vi "SUMMER SUNDAY BYTE[5].vi"() -> ()   [LabVIEW 2009]
uses:
  <vilib>/ULx/Create Channel.llb/ULx Create Channel (AI-Voltage-Basic).vi
  <vilib>/ULx/Create Channel.llb/ULx Create Channel (DO-Digital Output).vi
  <vilib>/ULx/Read.llb/ULx Read (Analog DBL 1Chan 1Samp).vi
  <vilib>/ULx/Write.llb/ULx Write (Digital Bool 1Line 1Point).vi
panel:
  out "Hutch Close":bool
  in  "Hutch Light":bool
  out "POWER":bool
  out "data":dbl format="%_6g"
  out "xray":bool caption="BitValue"
  out "ENERGY LEVEL":dbl(knob) scale=0.0..15.0
  out "Beam Pot":dbl format="%_6g"
  out "READY 2":bool
  out "DUMP":bool
  out "POWER":bool
  out "?":bool
  out "?":bool
  out "?":bool
  out "?":bool
  out "?":bool
  out "?":bool
  out "?":bool
  out "?":bool
  out "?":bool
  out "?":bool
  out "OPEN":bool
  out "CLOSED":bool
  out "READY":bool
  out "FAULT":bool
  out "MAGNET FORCE":dbl(slide) scale=0.0..10.0
  out "READY":bool
  out "TEMPERATURE":dbl(slide) scale=0.0..100.0
  in  "stop":bool
  out "?":bool
  out "?":bool
  out "?":bool
  out "?":bool
  out "FAULT":bool
  out "POWER":bool
  out "FLOW IN GPM":dbl(knob) scale=0.0..15.0
  # "USERS LAB AREA"
  # "BEAM STATUS"
  # "ROOM"
  # "XRAY"
  # "PUMP STATION"
  # "MAGNET STATUS"
  # "ORBIT"
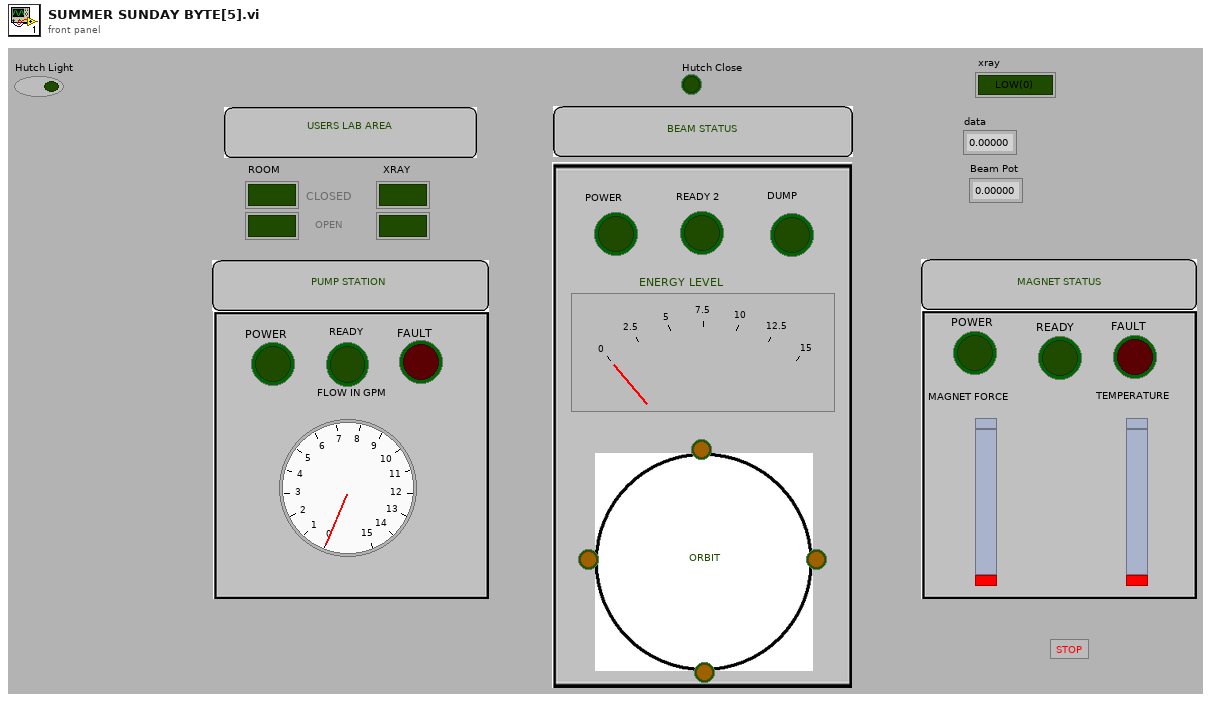
[diagram p1: front panel]
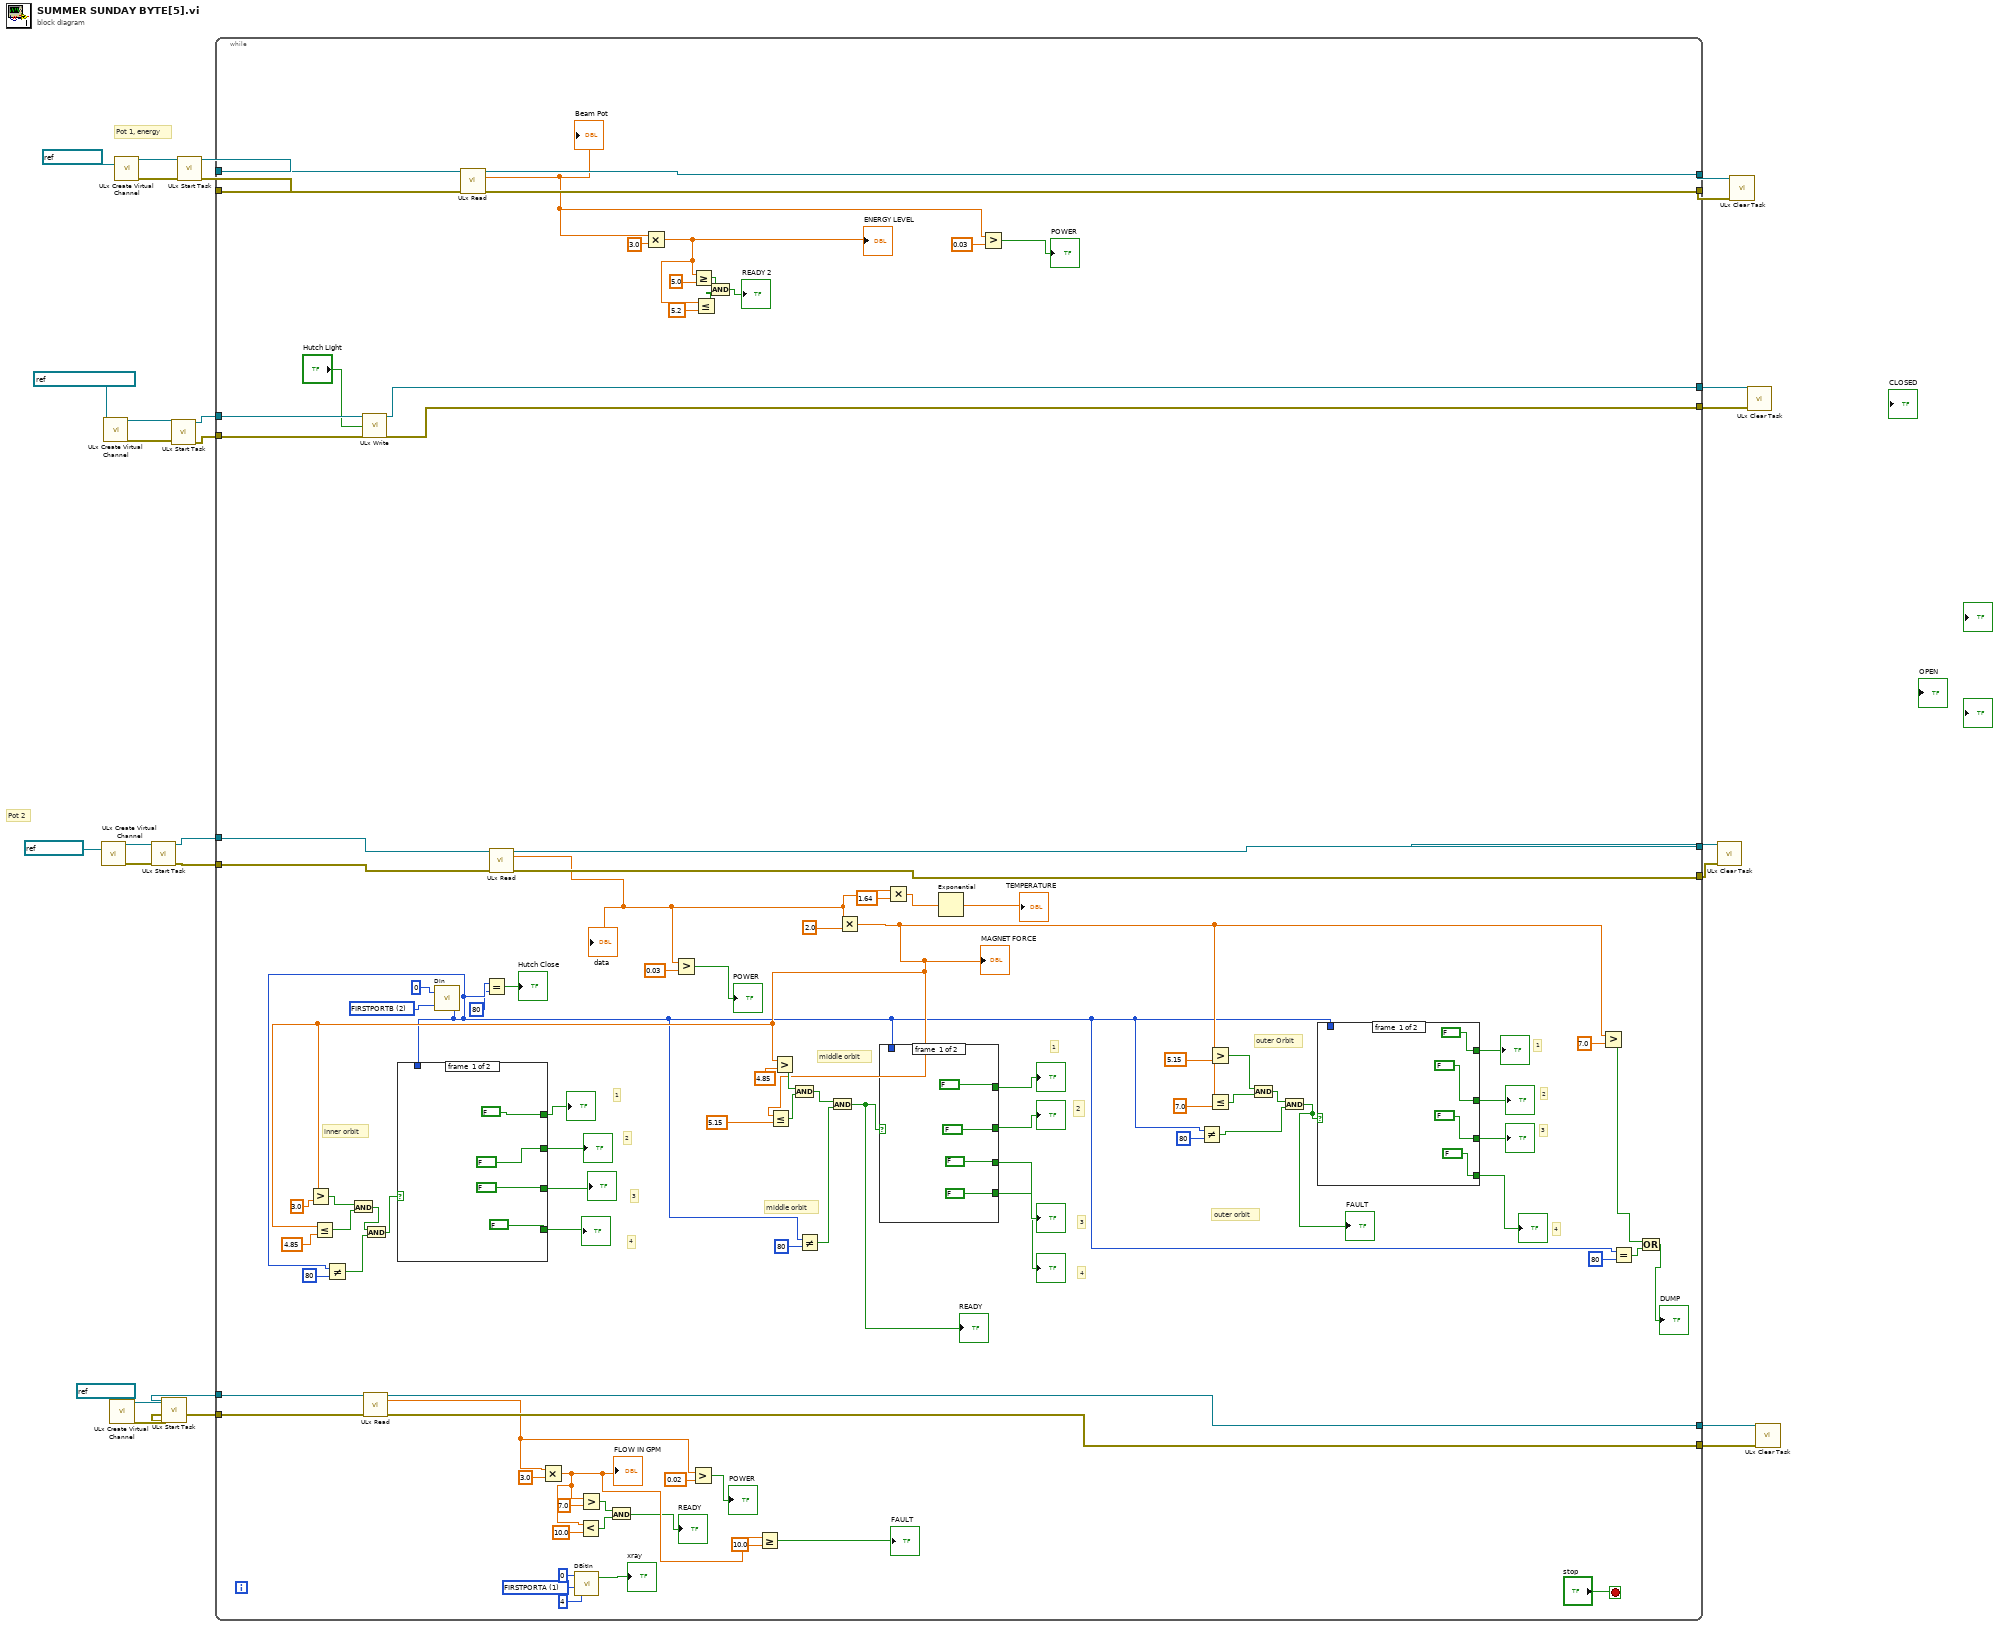
[diagram p0: block diagram]
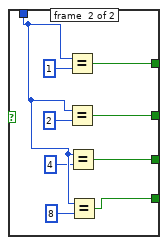
[diagram p2: hidden frame]
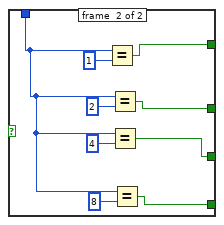
[diagram p3: hidden frame]
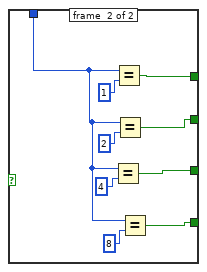
[diagram p4: hidden frame]
diagram:
  # "Pot 2"
  # "Pot 1, energy"
  n1 = call-poly <vilib>:"ULx Create Virtual Channel.vi"("physical channels"=refnum<k21> "Dev0/Ai1") -> ("task out"=w22:refnum<k24>, "error out"=w21:errorcluster)  [unwired: 13 in]
  n2 = call-poly <vilib>:"ULx Create Virtual Channel.vi"("lines"=refnum<k21> "Dev0/1stPortA/Do0") -> ("task out"=w7:refnum<k24>, "error out"=w6:errorcluster)  [unwired: 13 in]
  n3 = call-poly <vilib>:"ULx Create Virtual Channel.vi"("physical channels"=refnum<k21> "Dev0/Ai2") -> ("task out"=w14:refnum<k24>, "error out"=w13:errorcluster)  [unwired: 13 in]
  n4 = call-poly <vilib>:"ULx Create Virtual Channel.vi"("physical channels"=refnum<k21> "Dev0/Ai0") -> ("task out"=w28:refnum<k24>, "error out"=w27:errorcluster)  [unwired: 13 in]
  n5 = call <vilib>:"ULx Start Task.vi"("task in"=w22, "error in"=w21) -> ("task out"=w20:refnum<k24>, "error out"=w19:errorcluster)  [unwired: 12 in]
  n6 = call <vilib>:"ULx Start Task.vi"("task in"=w14, "error in"=w13) -> ("task out"=w12:refnum<k24>, "error out"=w11:errorcluster)  [unwired: 12 in]
  n7 = call <vilib>:"ULx Start Task.vi"("task in"=w7, "error in"=w6) -> ("task out"=w4:refnum<k24>, "error out"=w3:errorcluster)  [unwired: 12 in]
  n8 = call <vilib>:"ULx Start Task.vi"("task in"=w28, "error in"=w27) -> ("task out"=w26:refnum<k24>, "error out"=w25:errorcluster)  [unwired: 12 in]
  n9 = while {
    tunnel: w26 -> [w125]
    tunnel: w25 -> [w124]
    tunnel: [w123] -> w24
    tunnel: [w122] -> w23
    tunnel: w20 -> [w120]
    tunnel: w19 -> [w119]
    tunnel: [w118] -> w18
    tunnel: [w117] -> w17
    tunnel: w12 -> [w76]
    tunnel: w11 -> [w75]
    tunnel: [w74] -> w9
    tunnel: [w73] -> w8
    tunnel: w4 -> [w36]
    tunnel: w3 -> [w35]
    tunnel: [w34] -> w2
    tunnel: [w33] -> w1
    stop <- "stop" stop-if-true
    w71 = 1 items=["AUXPORT", "FIRSTPORTA"] ("PortType")
    w94 = 2 items=["AUXPORT", "FIRSTPORTA", "FIRSTPORTB", "FIRSTPORTCL", "FIRSTPORTCH", "SECONDPORTA", "SECONDPORTB", "SECONDPORTCL", "SECONDPORTCH", "THIRDPORTA", "THIRDPORTB", "THIRDPORTCL", "THIRDPORTCH", "FOURTHPORTA", "FOURTHPORTB", "FOURTHPORTCL", "FOURTHPORTCH", "FIFTHPORTA", "FIFTHPORTB", "FIFTHPORTCL", "FIFTHPORTCH", "SIXTHPORTA", "SIXTHPORTB", "SIXTHPORTCL", "SIXTHPORTCH", "SEVENTHPORTA", "SEVENTHPORTB", "SEVENTHPORTCL", "SEVENTHPORTCH", "EIGTHPORTA", "EIGHTHPORTB", "EIGHTHPORTCL", "EIGHTHPORTCH"] ("PortNum")
    # "outer Orbit"
    # "middle orbit"
    # "4"
    # "3"
    # "2"
    # "1"
    # "1"
    # "2"
    # "3"
    # "4"
    # "4"
    # "3"
    # "2"
    # "1"
    # "outer orbit"
    # "inner orbit"
    # "middle orbit"
    n10 = call-poly <vilib>:"ULx Write.vi"("task in"=w36, "data"="Hutch Light", "error in"=w35) -> ("task out"=w34:refnum<k24>, "error out"=w33:errorcluster)  [unwired: 10 in, 1 out]
    n11 = call-poly <vilib>:"ULx Read.vi"("task in"=w76, "error in"=w75) -> ("task out"=w74:refnum<k24>, "data"=w63:dbl, "error out"=w73:errorcluster)  [unwired: 11 in]
    n12 = call <menus>:"DIn.VI"("PortNum"=w94, "BoardNum"=u32 0) -> ("DataValue"=w31:i16)  [unwired: 1 out]
    n13 = Not Equal?(x=w31, y=i16 80) -> (x != y?=w104:bool)
    n14 = call-poly <vilib>:"ULx Read.vi"("task in"=w125, "error in"=w124) -> ("task out"=w123:refnum<k24>, "data"=w37:dbl, "error out"=w122:errorcluster)  [unwired: 11 in]
    "Beam Pot" <- w37
    n15 = Equal?(x=w31, y=i16 80) -> (x = y?=→"Hutch Close":bool)
    n16 = call-poly <vilib>:"ULx Read.vi"("task in"=w120, "error in"=w119) -> ("task out"=w118:refnum<k24>, "data"=w41:dbl, "error out"=w117:errorcluster)  [unwired: 11 in]
    "data" <- w41
    n17 = Multiply(x=w63, y=3.0) -> (x*y=w48:dbl)
    "FLOW IN GPM" <- w48
    n18 = call <menus>:"DBitIn.VI"("BitNum"=4, "PortType"=w71, "BoardNum"=u32 0) -> ("BitValue"=→"xray":bool)  [unwired: 1 out]
    n19 = Less?(x=w48, y=10.0) -> (x < y?=w46:bool)
    n20 = Greater?(x=w48, y=7.0) -> (0:w47:bool)
    n21 = And(x=w47, y=w46) -> (x .and. y?=→"READY":bool)
    n22 = Multiply(x=w37, y=3.0) -> (x*y=w58:dbl)
    "ENERGY LEVEL" <- w58
    n23 = Greater?(x=w41, y=0.03) -> (0:→"POWER":bool)
    n24 = Greater?(x=w63, y=0.02) -> (0:→"POWER":bool)
    n25 = Greater Or Equal?(x=w58, y=5.0) -> (x >= y?=w55:bool)
    n26 = Less Or Equal?(x=w58, y=5.2) -> (x <= y?=w54:bool)
    n27 = And(x=w55, y=w54) -> (x .and. y?=→"READY 2":bool)
    n28 = Greater Or Equal?(x=w48, y=10.0) -> (x >= y?=→"FAULT":bool)
    n29 = Not Equal?(x=w31, y=i16 80) -> (x != y?=w90:bool)
    n30 = Multiply(x=w41, y=2.0) -> (x*y=w97:dbl)
    "MAGNET FORCE" <- w97
    n31 = Greater?(x=w97, y=3.0) -> (0:w113:bool)
    n32 = Less Or Equal?(x=w97, y=4.85) -> (x <= y?=w114:bool)
    n33 = And(x=w113, y=w114) -> (x .and. y?=w106:bool)
    n34 = And(x=w106, y=w104) -> (x .and. y?=w105:bool)
    n35 = case shown="True" w105 {
      tunnel: [FALSE w160] -> w79
      tunnel: [FALSE w159] -> w80
      tunnel: [FALSE w158] -> w77
      tunnel: [FALSE w157] -> w78
      tunnel: w31 -> [_ w165]
      frame #0 {
      }
      frame #1 {
        n36 = Equal?(x=w165, y=i16 4) -> (x = y?=w158:bool)
        n37 = Equal?(x=w165, y=i16 1) -> (x = y?=w160:bool)
        n38 = Equal?(x=w165, y=i16 2) -> (x = y?=w159:bool)
        n39 = Equal?(x=w165, y=i16 8) -> (x = y?=w157:bool)
      }
    }
    "?" <- w80
    "?" <- w77
    "?" <- w78
    "?" <- w79
    n40 = Less Or Equal?(x=w97, y=5.15) -> (x <= y?=w110:bool)
    n41 = Greater?(x=w97, y=4.85) -> (0:w111:bool)
    n42 = And(x=w111, y=w110) -> (x .and. y?=w103:bool)
    n43 = And(x=w103, y=w90) -> (x .and. y?=w61:bool)
    "READY" <- w61
    n44 = case shown="True" w61 {
      tunnel: [FALSE w139] -> w89
      tunnel: [FALSE w138] -> w88
      tunnel: [FALSE w137] -> w87
      tunnel: [FALSE w136] -> w86
      tunnel: w31 -> [_ w135]
      frame #0 {
      }
      frame #1 {
        n45 = Equal?(x=w135, y=i16 1) -> (x = y?=w139:bool)
        n46 = Equal?(x=w135, y=i16 2) -> (x = y?=w138:bool)
        n47 = Equal?(x=w135, y=i16 4) -> (x = y?=w137:bool)
        n48 = Equal?(x=w135, y=i16 8) -> (x = y?=w136:bool)
      }
    }
    "?" <- w89
    "?" <- w88
    "?" <- w87
    "?" <- w86
    n49 = Multiply(x=w41, y=1.64) -> (x*y=w39:dbl)
    n50 = Exponential(1:w39) -> (0:→"TEMPERATURE":dbl)
    n51 = Greater?(x=w37, y=0.03) -> (0:→"POWER":bool)
    n52 = Not Equal?(x=w31, y=i16 80) -> (x != y?=w84:bool)
    n53 = Greater?(x=w97, y=5.15) -> (0:w108:bool)
    n54 = Less Or Equal?(x=w97, y=7.0) -> (x <= y?=w107:bool)
    n55 = And(x=w108, y=w107) -> (x .and. y?=w96:bool)
    n56 = And(x=w96, y=w84) -> (x .and. y?=w42:bool)
    "FAULT" <- w42
    n57 = case shown="True" w42 {
      tunnel: [FALSE w144] -> w101
      tunnel: [FALSE w145] -> w100
      tunnel: [FALSE w146] -> w99
      tunnel: [FALSE w147] -> w98
      tunnel: w31 -> [_ w152]
      frame #0 {
      }
      frame #1 {
        n58 = Equal?(x=w152, y=i16 1) -> (x = y?=w147:bool)
        n59 = Equal?(x=w152, y=i16 2) -> (x = y?=w146:bool)
        n60 = Equal?(x=w152, y=i16 4) -> (x = y?=w145:bool)
        n61 = Equal?(x=w152, y=i16 8) -> (x = y?=w144:bool)
      }
    }
    "?" <- w98
    "?" <- w99
    "?" <- w100
    "?" <- w101
    n62 = Greater?(x=w97, y=7.0) -> (0:w43:bool)
    n63 = Equal?(x=w31, y=i16 80) -> (x = y?=w81:bool)
    n64 = Or(x=w43, y=w81) -> (x .or. y?=→"DUMP":bool)
  }
  n65 = call <vilib>:"ULx Clear Task.vi"("task in"=w18, "error in"=w17) -> ()  [unwired: 13 in, 1 out]
  n66 = call <vilib>:"ULx Clear Task.vi"("task in"=w24, "error in"=w23) -> ()  [unwired: 13 in, 1 out]
  n67 = call <vilib>:"ULx Clear Task.vi"("task in"=w2, "error in"=w1) -> ()  [unwired: 13 in, 1 out]
  n68 = call <vilib>:"ULx Clear Task.vi"("task in"=w9, "error in"=w8) -> ()  [unwired: 13 in, 1 out]
